vi "CryoCon Curve Header.vi"(4 "Error In":errorcluster, 5 "Calibration (Empty gives dialog)":string, 6 "Sensor Type":T1, 7 "Sensor Number":u32 max=11 step=1) -> (0 "error out":errorcluster, 1 "Header Array":string[](array[string]), 2 "Resistance":dbl[](array[numeric]), 3 "Temperature":dbl[](array[numeric]))   [LabVIEW 2020]
uses:
  Sub Controls/CryoCon Sensor Type.ctl
  <vilib>/Analysis/baseanly.llb/Mean (DBL).vi
  <vilib>/Analysis/2dsp.llb/Derivative x(t).vi
  <vilib>/Analysis/NI_AALPro.lvlib
  <vilib>/Analysis/NI_AALBase.lvlib
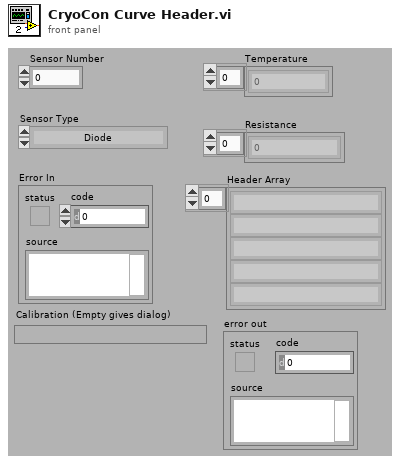
[diagram p1: front panel]
types:
  T1 = typedef "CryoCon Sensor Type.ctl" = enum16{"Diode", "AC Resistance", "DC Resistance 3.1 k½", "DC Resistance 312 ½", "DC Resistance 625 ½"}
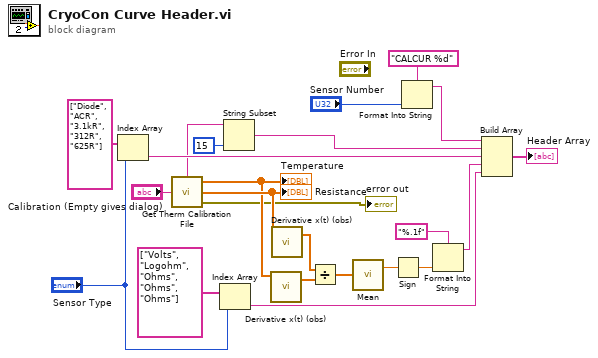
[diagram p0: block diagram]
diagram:
  n1 = Index Array(array=string[] ["Diode", "ACR", "3.1kR", "312R", "625R"], index="Sensor Type") -> (element=w11:string)
  n2 = call "Get Therm Calibration File.vi"("Calibration (Empty gives dialog)"="Calibration (Empty gives dialog)") -> ("Calbration Name"=w10:string, "Temperature"=w12:dbl[], "Resistance"=w13:dbl[], "error out"=→"error out":errorcluster)
  "Resistance" <- w13
  "Temperature" <- w12
  n3 = Index Array(array=string[] ["Volts", "Logohm", "Ohms", "Ohms", "Ohms"], index="Sensor Type") -> (element=w4:string)
  n4 = String Subset(string=w10, length (rest)=15 ("length (rest)")) -> (substring=w3:string)  [unwired: 1 in]
  n5 = call <vilib>:"Derivative x(t) (obs).vi"("X"=w12) -> ("dX/dt"=w15:dbl[])  [unwired: 3 in, 1 out]
  n6 = call <vilib>:"Derivative x(t) (obs).vi"("X"=w13) -> ("dX/dt"=w14:dbl[])  [unwired: 3 in, 1 out]
  n7 = Divide(x=w14, y=w15) -> (x/y=w16:dbl[])
  n8 = call-poly <vilib>:"Mean.vi"("X"=w16) -> ("mean"=w17:dbl)  [unwired: 1 out]
  n9 = Sign(1:w17) -> (0:w18:dbl)
  n10 = Format Into String(format string="CALCUR %d" ("Format String"), "Sensor Number") -> (resulting string=w23:string)  [unwired: 2 in, 1 out]
  n11 = Format Into String(format string="%.1f", w18) -> (resulting string=w5:string)  [unwired: 2 in, 1 out]
  n12 = Build Array(w23, w3, w11, w5, w4) -> (→"Header Array":string[])
